vi "Get Cluster Element Index.vi"(9 "Element Name":string, 11 "Cluster":variant) -> (3 "Element Index":i32)   [LabVIEW 2011]
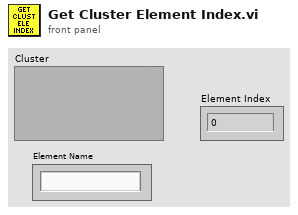
[diagram p1: front panel]
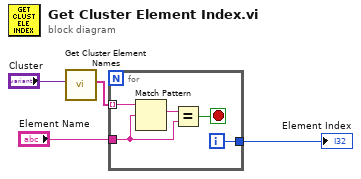
[diagram p0: block diagram]
diagram:
  n1 = call "Get Cluster Element Names.vi"("Cluster"="Cluster") -> ("Element Names"=w4:string[])  [unwired: 9 in, 1 out]
  n2 = for {
    tunnel: w4 -> [w9] mode=indexing
    tunnel: "Element Name" -> [w7]
    tunnel: [w5] -> w2
    i -> [w5]
    stop <- w6 stop-if-true
    n3 = Match Pattern(string=w9, regular expression=w7) -> (match substring=w8:string)  [unwired: 1 in, 3 out]
    n4 = Equal?(x=w8, y=w7) -> (x = y?=w6:bool)
  }
  "Element Index" <- w2
